vi "Com_SECS Equipment _Stream_S7F2.vi"(8 "error in":errorcluster, 11 "Process Program Status(PPGNT)":T1(ring)) -> (0 "error out":errorcluster, 3 "SECS Packet":T2)   [LabVIEW 2016]
uses:
  Data Def/Com_SECS Equipment _SECS Packet.ctl
  Data Def/Com_SECS Equipment _Message Type.ctl
  Data Def/Com_SECS Equipment _Protocol Type.ctl
  Data Def/Com_SECS Equipment _Stream Type.ctl
  Data Def/Com_SECS Equipment _Build Message Setting.ctl
  Data Message/Com_SECS Equipment _Data Message_Binary.vi
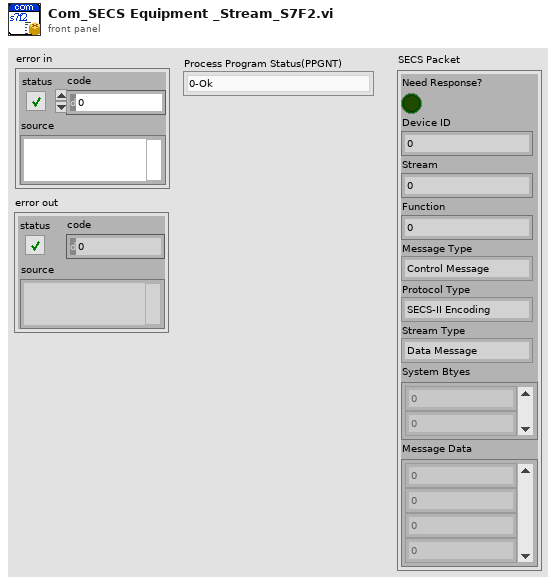
[diagram p1: front panel]
types:
  T1 = enum8{"0-Ok", "1-already have", "2-no space", "3-invalid PPID", "4-busy,try later", "5-will not accept", "6-other error"}
  T2 = typedef "Com_SECS Equipment _SECS Packet.ctl" = cluster{"Need Response?":bool, "Device ID":u16, "Stream":u8, "Function":u8, "Message Type":T3, "Protocol Type":T4, "Stream Type":T5, "System Btyes":u8[], "Message Data":u8[]}
  T3 = typedef "Com_SECS Equipment _Message Type.ctl" = enum16{"Control Message", "Data Message"}
  T4 = typedef "Com_SECS Equipment _Protocol Type.ctl" = enum16{"SECS-II Encoding", "Reserved"}
  T5 = typedef "Com_SECS Equipment _Stream Type.ctl" = enum16{"Data Message", "Select.req", "Select.rsp", "Deselect.req", "Deselect.rsp", "Linktest.req", "Linktest.rsp", "Reject.req", "Separate.req", "Reserve"}
  T6 = typedef "Com_SECS Equipment _Build Message Setting.ctl" = cluster{"Stream":u8, "Function":u8, "Need Response?":bool}
  T7 = typedef "Com_SECS Equipment _Message Data.ctl" = cluster{"Index":i32, "Data Item Format":T8, "Format Code":T9, "Parent Index":i32, "Child Index":i32[], "Data":variant}
  T8 = typedef "Com_SECS Equipment _Data Item Format.ctl" = enum16{"Data Type", "Value"}
  T9 = typedef "Com_SECS Equipment _Format Code.ctl" = enum16{"L", "A", "B", "Boolean", "J", "I1", "I2", "I4", "I8", "U1", "U2", "U4", "U8", "F4", "F8", "Char"}
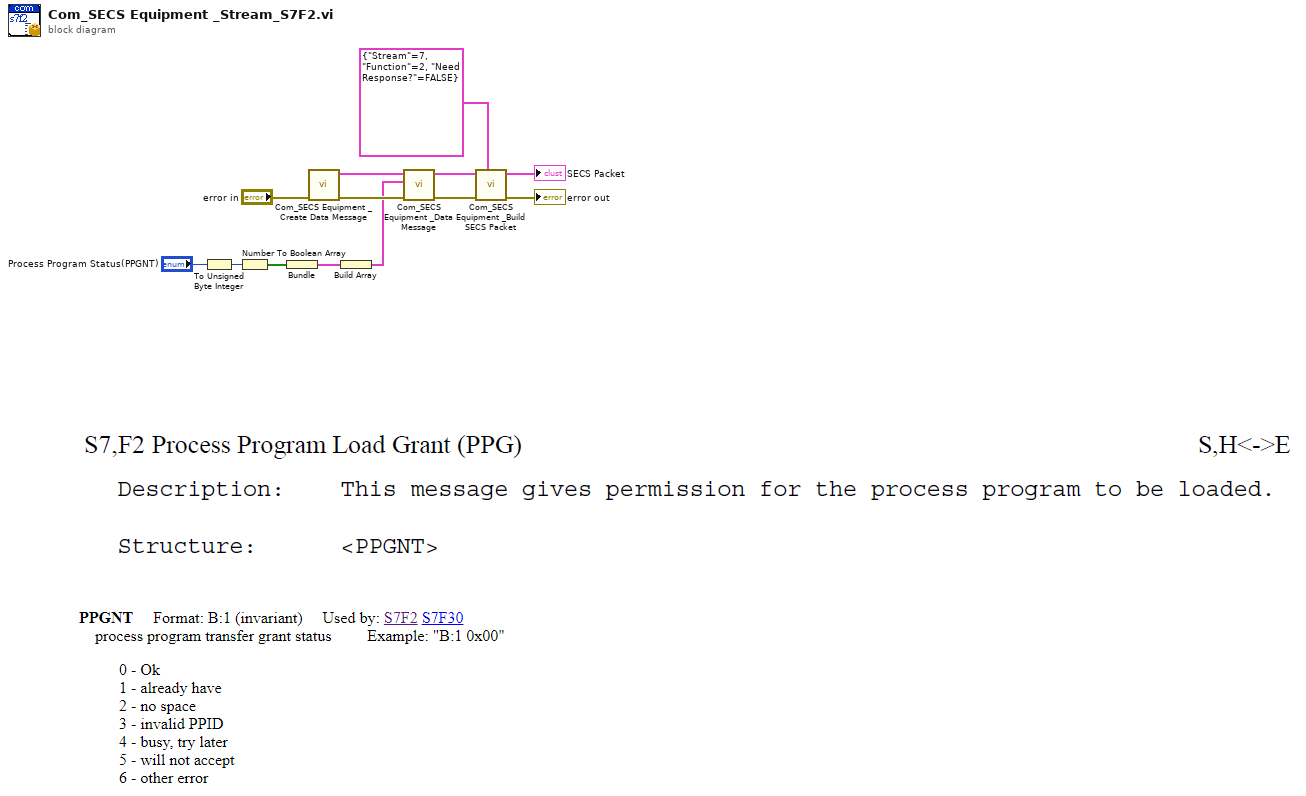
[diagram p0: block diagram]
diagram:
  n1 = To Unsigned Byte Integer(number="Process Program Status(PPGNT)") -> (unsigned 8bit integer=w6:u8)
  n2 = Number To Boolean Array(number=w6) -> (Boolean array=w5:bool[])
  n3 = Bundle("Boolean array"=w5) -> (w4:cluster{"Boolean array":bool[]})  [unwired: 1 in]
  n4 = call "Com_SECS Equipment _Create Data Message.vi"("error in"="error in") -> ("error out"=w8:errorcluster, "Message Data"=w9:T7[])  [unwired: 9 in]
  n5 = Build Array(w4) -> (w3:cluster{"Boolean array":bool[]}[])
  n6 = call-poly "Com_SECS Equipment _Data Message.vi"("error in"=w8, "Data Cluster"=w3, "Message Data In"=w9) -> ("error out"=w2:errorcluster, "Message Data Out"=w1:T7[])  [unwired: 7 in]
  n7 = call "Com_SECS Equipment _Build SECS Packet.vi"("Build Message Setting"=T6 {"Stream"=7, "Function"=2, "Need Response?"=FALSE}, "error in"=w2, "Message Data"=w1) -> ("error out"=→"error out":errorcluster, "SECS Packet"=→"SECS Packet":T2)  [unwired: 7 in]
